vi "example.vi"() -> ()   [LabVIEW 2013]
uses:
  test displayable.lvclass
  properties.ctl
  test displayable.lvclass/test displayable.ctl
  Write 1.vi
  Read 2.vi
  Write 2.vi
  set value.vi
  displayable.lvclass
panel:
  out "error out":errorcluster
  out "2ind":dbl
  in  "stop":bool
  out "ind":dbl
  in  "ctl":dbl
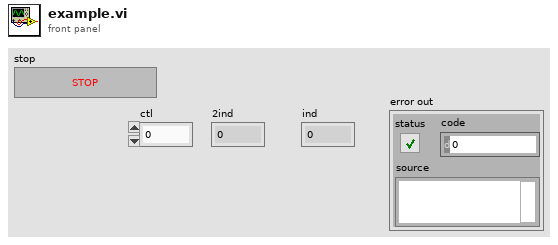
[diagram p1: front panel]
types:
  T1 = typedef "test displayable.lvclass/properties.ctl" = enum16{"1", "2"}
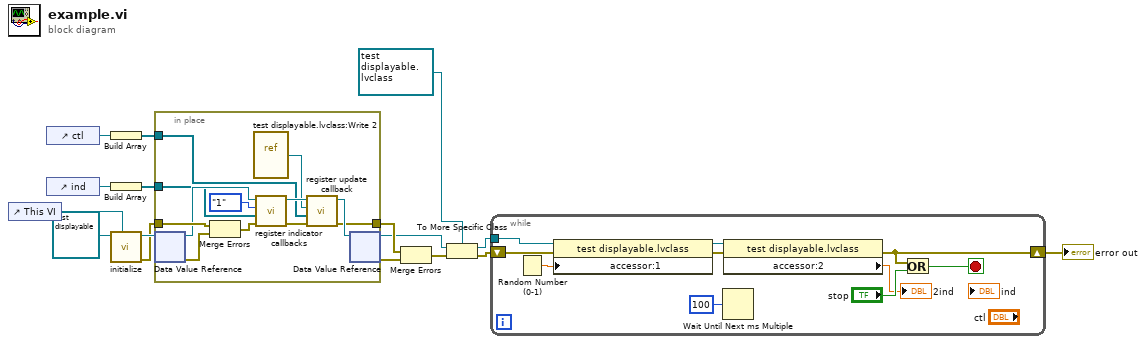
[diagram p0: block diagram]
diagram:
  n1 = control-ref of="This VI"() -> (w1:refnum<vi>)
  n2 = control-ref of="ctl"() -> (w9:refnum<vi>)
  n3 = control-ref of="ind"() -> (w13:refnum<vi>)
  n4 = Build Array(w9) -> (w8:refnum<vi>[])
  n5 = Build Array(w13) -> (w12:refnum<vi>[])
  n6 = call "initialize.vi"("VI Refnum"=w1, "displayable in"=refnum<class "test displayable.lvclass"> refnum ("test displayable.lvclass")) -> ("error out"=w14:errorcluster, "displayable"=w15:refnum<data-value>)  [unwired: 8 in]
  n7 = in-place {
    in-place-border: w14 -> [w28]
    in-place-border: w12 -> [w24]
    in-place-border: [w20] -> w11
    in-place-border: w8 -> [w18]
    n8 = in-place-dvr #1(w15) -> (w25:refnum<class "displayable.lvclass">, w26:errorcluster)
    n9 = Merge Errors(w28, w26) -> (w27:errorcluster)
    n10 = vi-ref "test displayable.lvclass:Write 2.vi"() -> (w17:refnum<vi>)
    n11 = call "register indicator callbacks.vi"("error in"=w27, "controls"=w24, "value index"=properties."1" ("props"), "displayable in"=w25) -> ("error out"=w19:errorcluster, "displayable out"=w22:refnum<class "displayable.lvclass">)  [unwired: 6 in]
    n12 = call "register update callback.vi"("error in"=w19, "controls"=w18, "VI Refnum"=w17, "displayable in"=w22) -> ("error out"=w20:errorcluster, "displayable out"=w21:refnum<class "displayable.lvclass">)  [unwired: 6 in]
    n13 = in-place-dvr #1(w21) -> (w5:refnum<data-value>, w10:errorcluster)
  }
  n14 = Merge Errors(w11, w10) -> (w7:errorcluster)
  n15 = To More Specific Class(target class=refnum<data-value> refnum, reference=w5, error in=w7) -> (specific class reference=w4:refnum<data-value>, error out=w6:errorcluster)
  n16 = while {
    shift-right: [w30] -> w2
    shift-left: w6 -> [w37]
    tunnel: w4 -> [w36]
    stop <- w31 stop-if-true
    n17 = Random Number (0-1)() -> (number: 0 to 1=w35:dbl)
    n18 = property class="test displayable.lvclass"(reference=w36, error in=w37, "accessor:1"=w35) -> (reference out=w34:refnum<data-value>, error out=w33:errorcluster)
    n19 = Wait Until Next ms Multiple(millisecond multiple=u32 100) -> ()  [unwired: 1 out]
    n20 = property class="test displayable.lvclass"(reference=w34, error in=w33) -> (error out=w30:errorcluster, "accessor:2"=→"2ind":dbl)  [unwired: 1 out]
    n21 = Or(x=w30, y="stop") -> (x .or. y?=w31:bool)
  }
  "error out" <- w2
